vi "write to fifo.vi"(0 "5785_3.2GHz_one channel in":refnum<class "5785_3.2GHz_one channel.lvclass">, 11 "error in (no error)":errorcluster) -> (4 "5785_3.2GHz_one channel out":refnum<class "5785_3.2GHz_one channel.lvclass">, 6 "done write file":bool=TRUE, 8 "num of pulses sent to the FPGA":u32, 10 "room on fifo":bool=TRUE, 15 "error out":errorcluster)   [LabVIEW 2021, in "5785_3.2GHz_one channel.lvclass"]
uses:
  5785_3.2GHz_one channel.lvclass
  5785_3.2GHz_one channel.lvclass/5785_3.2GHz_one channel.ctl
  <vilib>/Utility/error.llb/Error Cluster From Error Code.vi
  <vilib>/rvi/errors/niLvFpgaAdjustHostInterfaceError.vi
  <vilib>/rvi/interface/nirviMethod/nirviMethod.xnode
  <vilib>/FPGAPlugInAG/Dynamic/niLvFpga_WriteFifo_Dynamic.vi
  <vilib>/rvi/errors/niLvFpgaMergeErrorWithErrorCode.vi
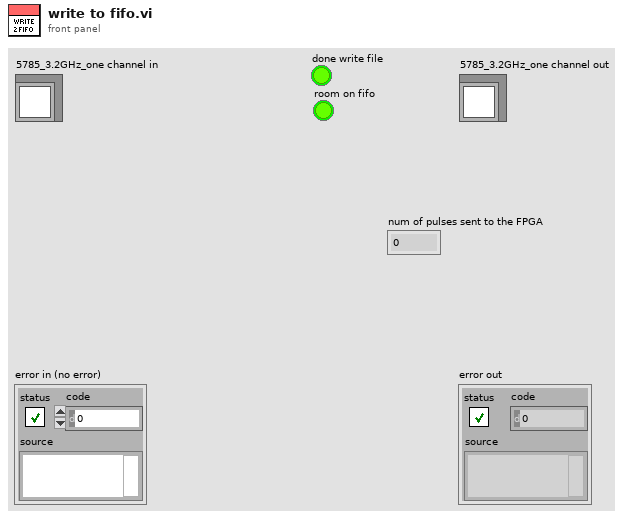
[diagram p1: front panel]
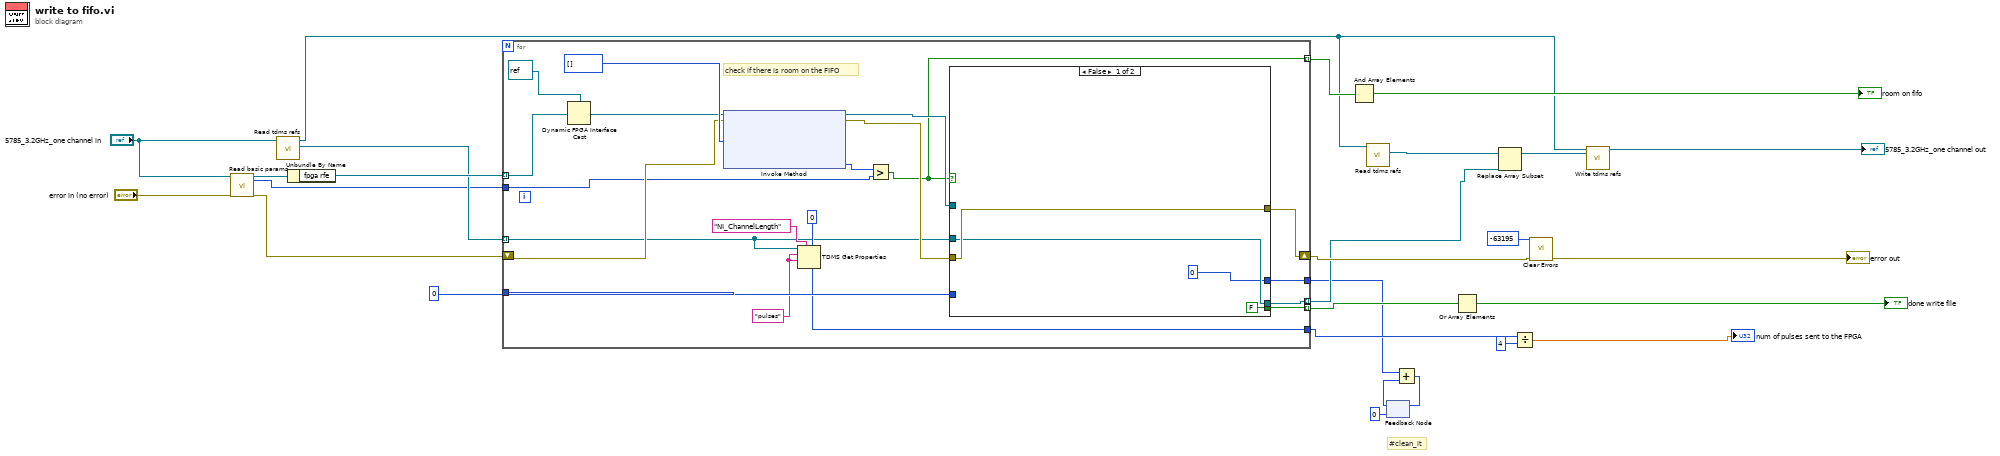
[diagram p0: block diagram]
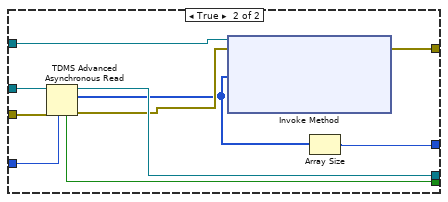
[diagram p2: hidden frame]
diagram:
  # "#clean_it"
  n1 = call-dynamic "Read basic params.vi"("device_type in"="5785_3.2GHz_one channel in", "error in (no error)"="error in (no error)") -> ("device_type out"=w14:refnum<class "5785_3.2GHz_one channel.lvclass">, "buffer size"=w16:u32, "error out"=w12:errorcluster)  [unwired: 12 in, 3 out]
  n2 = call-dynamic "Read tdms refs.vi"("device_type in"="5785_3.2GHz_one channel in") -> ("tdms refs"=w17:refnum<k34>[], "device_type out"=w10:refnum<class "5785_3.2GHz_one channel.lvclass">)  [unwired: 8 in, 1 out]
  n3 = Unbundle By Name(w14) -> ("fpga rfe"=w25:refnum<k20>[])
  n4 = for {
    tunnel: w17 -> [w30] mode=indexing
    tunnel: w25 -> [w36] mode=indexing
    tunnel: u64 0 ("type") -> [w47]
    tunnel: [w46] -> w26 mode=indexing
    tunnel: [w45] -> w21 mode=indexing
    shift-right: [w44] -> w23
    shift-left: w12 -> [w42]
    tunnel: w16 -> [w41]
    tunnel: [w38] -> w22 mode=indexing
    tunnel: [w29] -> w7
    tunnel: [w28] -> w4
    w31 = "pulses" ("channel name")
    # "check if there is room on the FIFO"
    n5 = Dynamic FPGA Interface Cast(Session In=refnum<k20> refnum ("FPGA VI Reference Out"), Type=w36) -> (Session Out=w35:refnum<k20>)
    n6 = xnode "Invoke Method"("FPGA VI Reference In"=w35, "error in"=w42, "Data"=u64[] []) -> ("FPGA VI Reference Out"=w39:refnum<k20>, "error out"=w40:errorcluster, "Empty Elements Remaining"=w37:u32)  [unwired: 1 in]
    n7 = TDMS Get Properties(5:u64 0, 7:"NI_ChannelLength" ("property name"), 9:w31, 10:w31, 11:w30) -> (4:w29:u64)  [unwired: 1 in, 5 out]
    n8 = Greater?(x=w37, y=w41) -> (0:w38:bool)
    n9 = case shown="False" w38 {
      tunnel: w30 -> [w50 w61]
      tunnel: w47 -> [_ w60]
      tunnel: [FALSE ("read process finished?") w59] -> w46
      tunnel: [w50 w58] -> w45
      tunnel: [w51 w56] -> w44
      tunnel: w40 -> [w51 w55]
      tunnel: w39 -> [_ w54]
      tunnel: [0 w52] -> w28
      frame False {
      }
      frame True {
        n10 = TDMS Advanced Asynchronous Read(6:w60, 8:w55, 11:w61) -> (0:w57:errorcluster, 2:w53:u64[], 3:w58:refnum<k34>, 4:w59:bool)
        n11 = xnode "Invoke Method"("FPGA VI Reference In"=w54, "error in"=w57, "Data"=w53) -> ("error out"=w56:errorcluster)  [unwired: 1 in, 2 out]
        n12 = Array Size(array=w53) -> (size(s)=w52:i32)
      }
    }
  }
  n13 = And Array Elements(Boolean array=w22) -> (logical AND=→"room on fifo":bool)
  n14 = call-dynamic "Read tdms refs.vi"("device_type in"=w10) -> ("tdms refs"=w11:refnum<k34>[])  [unwired: 8 in, 2 out]
  n15 = feedback #1(0) -> (w3:i32)
  n16 = Add(x=w4, y=w3) -> (x+y=w2:i32)
  n17 = feedback-in #1(w2) -> ()
  n18 = Or Array Elements(Boolean array=w26) -> (logical OR=→"done write file":bool)
  n19 = Replace Array Subset(array=w11, new element=w21) -> (w8:refnum<k34>[])  [unwired: 1 in]
  n20 = Divide(x=w7, y=u64 4) -> (x/y=→"num of pulses sent to the FPGA":dbl)
  n21 = call <vilib>:"Clear Errors.vi"("error in (no error)"=w23, "specific error code to clear (0: all)"=-63195) -> ("error out"=→"error out":errorcluster)  [unwired: 4 in, 1 out]
  n22 = call-dynamic "Write tdms refs.vi"("tdms refs"=w8, "device_type in"=w10) -> ("device_type out"=→"5785_3.2GHz_one channel out":refnum<class "5785_3.2GHz_one channel.lvclass">)  [unwired: 8 in, 1 out]
